vi "Run Script.vi"(8 "error in (no error)":errorcluster, 9 "Script Variable":string, 10 "Script Type (0: Specified Script)":i32(ring) items=["Specified Script", "Anonymous Script."], 11 "VISA resource name":refnum<visa-resource-name>) -> (0 "error out":errorcluster, 3 "VISA resource name out":refnum<visa-resource-name>)   [LabVIEW 2015, in "Keithley 2600 Series.lvlib"]
doc: "Runs a script.\n\n<b>Note:</b>\nWhen you run a script that contains the command of \"print()\", you need to call the <b>Print Variable </b>VI and set the variable name to \"Nil\" to read the output data or message."
uses:
  Keithley 2600 Series.lvlib
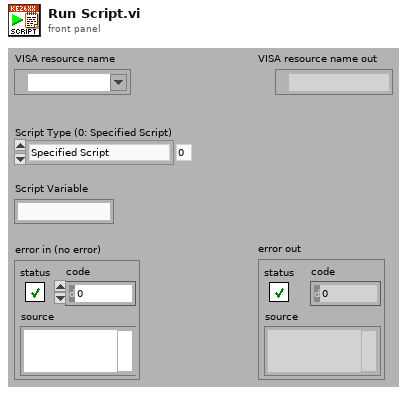
[diagram p1: front panel]
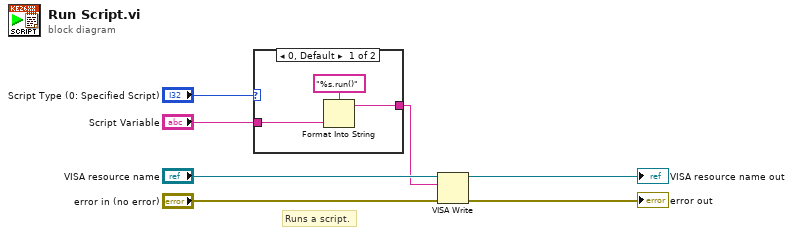
[diagram p0: block diagram]
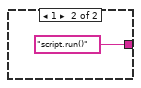
[diagram p2: hidden frame]
diagram:
  # "Runs a script."
  n1 = case shown="0, Default" "Script Type (0: Specified Script)" {
    tunnel: "Script Variable" -> [w9 _]
    tunnel: [w8 "script.run()"] -> w3
    frame 0, Default {
      n2 = Format Into String(format string="%s.run()", w9) -> (resulting string=w8:string)  [unwired: 2 in, 1 out]
    }
    frame 1 {
    }
  }
  n3 = VISA Write(VISA resource name="VISA resource name", write buffer=w3, error in (no error)="error in (no error)") -> (VISA resource name out=→"VISA resource name out":refnum<visa-resource-name>, error out=→"error out":errorcluster)  [unwired: 1 out]
